vi "StageRotate.vi"(0 "Axis":T1={"Serial port handle"="", "Axis"="", "Controller #"=0, "Min position"=0.0, "Max position"=0.0, "Min velocity"=0.0, "Max velocity"=0.0, "Firmware"="", "Device ID"=0, "Variable event"=refnum, "Variable ref"=refnum, "Resolution, usteps/step"=0, "Serial port semaphore"=refnum, "Joystick buttons"={"MinDir"=1, "MaxDir"=2, "MedSpeed"=5, "HighSpeed"=6}} {"Joystick buttons"."HighSpeed" min=1 max=25 step=1; "Joystick buttons"."MedSpeed" min=1 max=25 step=1; "Joystick buttons"."MaxDir" min=1 max=25 step=1; "Joystick buttons"."MinDir" min=1 max=25 step=1}, 2 "Joystick event":T4, 3 "Stop event":refnum<user-event>, 5 "error in":errorcluster={"status"=FALSE, "code"=1073676294, "source"="VISA Read in Zaber TLCM.lvclass:Command.vi:1820008->Zaber TLCM.lvclass:Get home position.vi->Zaber TLCM.lvclass:Get limits.vi->Zaber TLCM.lvclass:Join.vi->Swan probe.vi"}) -> (14 "Axis out":T1={"Serial port handle"="", "Axis"="", "Controller #"=0, "Min position"=0.0, "Max position"=0.0, "Min velocity"=0.0, "Max velocity"=0.0, "Firmware"="", "Device ID"=0, "Variable event"=refnum, "Variable ref"=refnum, "Resolution, usteps/step"=0, "Serial port semaphore"=refnum, "Joystick buttons"={"MinDir"=1, "MaxDir"=2, "MedSpeed"=5, "HighSpeed"=6}} {"Joystick buttons"."HighSpeed" min=1 max=25 step=1; "Joystick buttons"."MedSpeed" min=1 max=25 step=1; "Joystick buttons"."MaxDir" min=1 max=25 step=1; "Joystick buttons"."MinDir" min=1 max=25 step=1}, 19 "error out":errorcluster)   [LabVIEW 2017]
uses:
  Joystick events/Joystick event.ctl
  GenericDataEvent/GenericEvent.ctl
  Zaber.ctl
  ZaberVariables.ctl
panel:
  out "JoystickValue":i16
  in  "Readback loop":bool
  in  "JoyHighVelocity":i32=6 caption="Max direction" min=1 max=25 step=1
  in  "JoyMediumVelocity":i32=5 caption="Max direction" min=1 max=25 step=1
  in  "JoyMaxDirection":i32=2 caption="Max direction" min=1 max=25 step=1
  in  "JoyMinDirection":i32=1 caption="Min direction" min=1 max=25 step=1
  in  "JoyHighVel":dbl=3.0 caption="High velocity, deg/s" min=1e-07 max=25.0 step=0.01 format="%#.4f"
  in  "JoyMediumVel":dbl=1.0 caption="Medium velocity, deg/s" min=1e-07 max=25.0 step=0.01 format="%#.4f"
  in  "JoyLowVel":dbl=0.02 caption="Low velocity, deg/s" min=1e-07 max=25.0 step=0.01 format="%#.4f"
  out "Name":string
  in  "VelocitySp":dbl=0.19998779296875002 caption="Velocity, deg/s" min=0.0 max=25.40003175 format="%#.6f"
  out "VelocityRb":dbl=0.19998779296875002 caption="X position" min=0.0 max=25.0 format="%#.6f"
  in  "PositionSp":dbl caption="Position, deg" min=0.0 max=25.40003175 format="%#.6f"
  in  "MaxSoftPosition":dbl=101.60003175000001 caption="Max soft position, deg" min=0.0 max=25.40003175 format="%#.4f"
  in  "MinSoftPosition":dbl caption="Min soft position, deg" min=0.0 max=25.40003175 format="%#.4f"
  out "PositionRb":dbl=0.8111490000000001 caption="X position" min=0.0 max=25.0 format="%#.6f"
  out "MaxVelocity":dbl=26.0 caption="Max velocity, deg/s" format="%#.4f"
  out "MaxPositionRb":dbl=101.60003175000001 caption="Max position, deg" format="%#.4f"
  out "MinPositionRb":dbl caption="Min position, deg" format="%#.4f"
  # "Joystick"
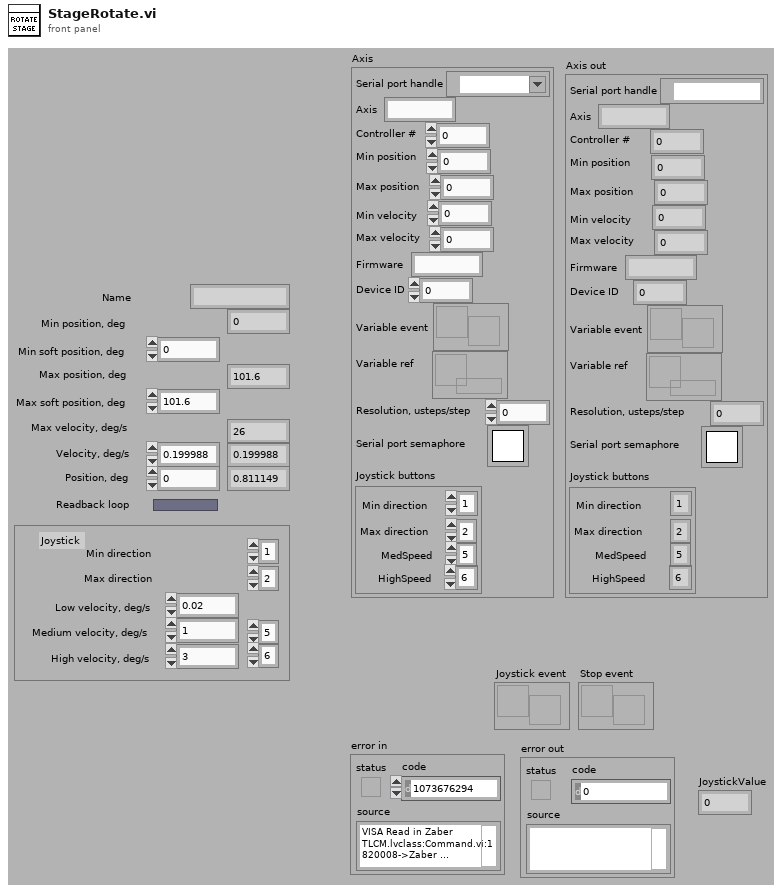
[diagram p1: front panel]
types:
  T1 = typedef "Zaber.ctl" = cluster{"Serial port handle":refnum<visa-resource-name>, "Axis":string, "Controller #":u8, "Min position":dbl, "Max position":dbl, "Min velocity":dbl, "Max velocity":dbl, "Firmware":string, "Device ID":i32, "Variable event":T2, "Variable ref":refnum<data-value>, "Resolution, usteps/step":i32, "Serial port semaphore":T3, "Joystick buttons":cluster{"MinDir":i32, "MaxDir":i32, "MedSpeed":i32, "HighSpeed":i32}}
  T2 = typedef "GenericEvent.ctl" = refnum<user-event>
  T3 = typedef "Semaphore RefNum" = refnum<k1>
  T4 = typedef "Joystick event.ctl" = refnum<user-event>
  T5 = cluster{"MinDir":i32, "MaxDir":i32, "MedSpeed":i32, "HighSpeed":i32}
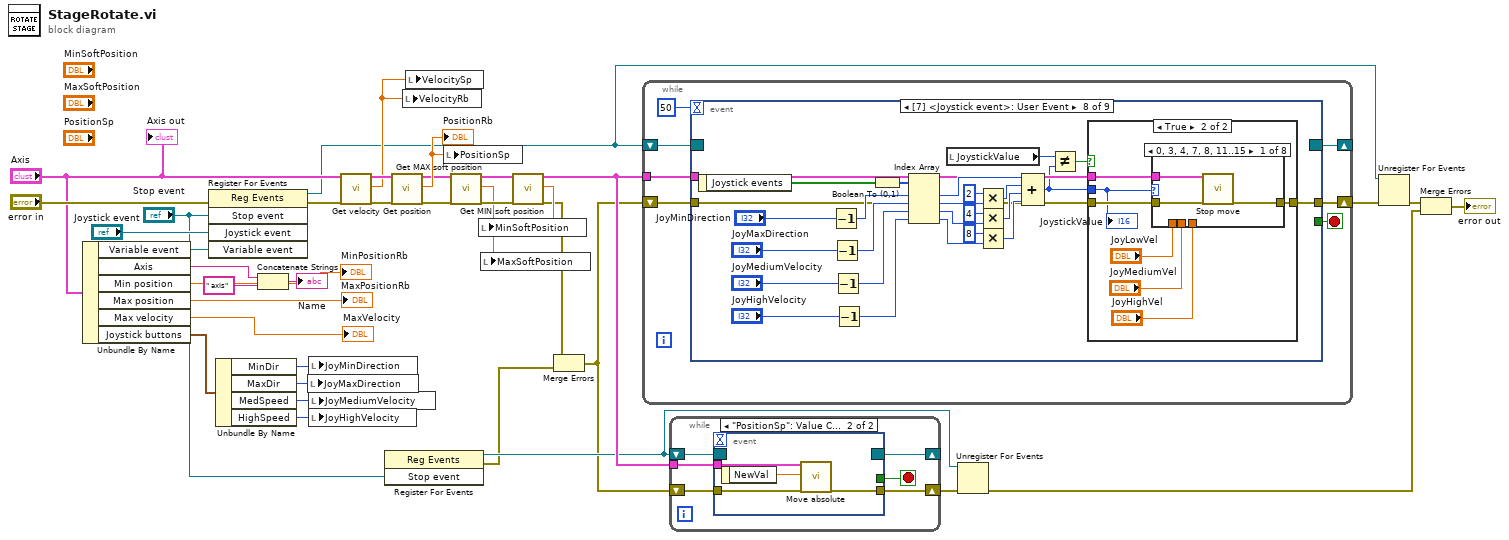
[diagram p0: block diagram]
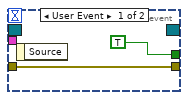
[diagram p2: hidden frame]
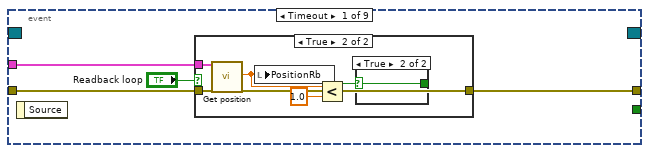
[diagram p3: hidden frame]
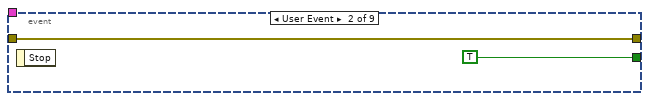
[diagram p6: hidden frame]
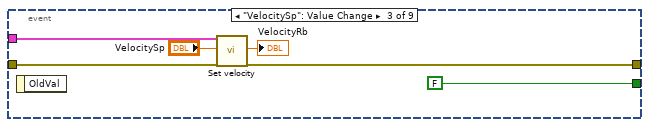
[diagram p7: hidden frame]
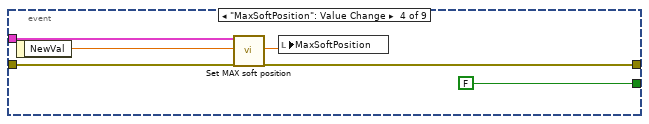
[diagram p8: hidden frame]
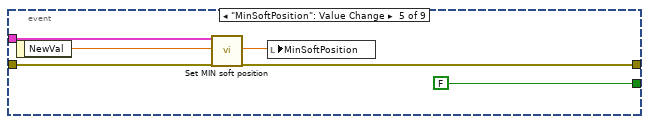
[diagram p9: hidden frame]
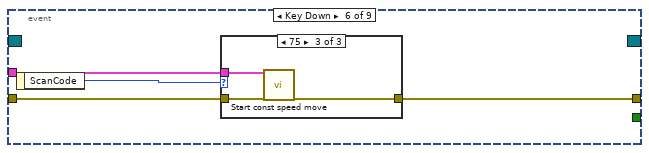
[diagram p10: hidden frame]
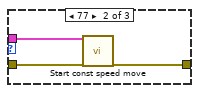
[diagram p12: hidden frame]
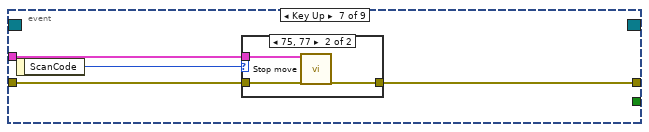
[diagram p13: hidden frame]
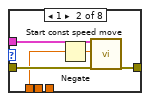
[diagram p16: hidden frame]
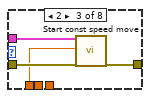
[diagram p17: hidden frame]
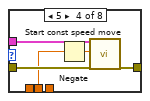
[diagram p18: hidden frame]
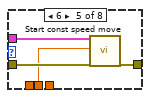
[diagram p19: hidden frame]
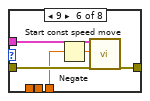
[diagram p20: hidden frame]
diagram:
  n1 = Unbundle By Name("Axis") -> ("Variable event"=w35:T2, "Axis"=w33:string, "Min position"=→"MinPositionRb":dbl, "Max position"=→"MaxPositionRb":dbl, "Max velocity"=→"MaxVelocity":dbl, "Joystick buttons"=w1:T5)
  n2 = register-events(error in="error in", "Stop event", "Joystick event", w35) -> (reference out=w11:refnum<event-registration>, error out=w27:errorcluster)  [unwired: 1 in]
  n3 = Unbundle By Name(w1) -> ("MinDir"=w16:i32, "MaxDir"=w15:i32, "MedSpeed"=w14:i32, "HighSpeed"=w13:i32)
  n4 = Concatenate Strings(w33, " axis" ("string")) -> (→"Name":string)
  n5 = local write "JoyMaxDirection"(w15) -> ()
  n6 = local write "JoyMinDirection"(w16) -> ()
  n7 = local write "JoyMediumVelocity"(w14) -> ()
  n8 = local write "JoyHighVelocity"(w13) -> ()
  n9 = call "Get velocity.vi"("Zaber"="Axis", "error in"=w27) -> ("Zaber out"=w31:T1, "Velocity, mm/s"=w30:dbl, "error out"=w38:errorcluster)  [unwired: 14 in, 1 out]
  n10 = register-events("Stop event") -> (reference out=w9:refnum<event-registration>, error out=w4:errorcluster)  [unwired: 2 in]
  n11 = call "Get position.vi"("Zaber"=w31, "error in"=w38) -> ("Zaber out"=w20:T1, "PositionRb"=w29:dbl, "error out"=w21:errorcluster)  [unwired: 13 in, 2 out]
  "PositionRb" <- w29
  n12 = local write "VelocityRb"(w30) -> ()
  n13 = local write "VelocitySp"(w30) -> ()
  n14 = local write "PositionSp"(w29) -> ()
  n15 = call "Get MAX soft position.vi"("Zaber"=w20, "error in"=w21) -> ("Zaber out"=w22:T1, "Max soft position"=w18:dbl, "error out"=w23:errorcluster)  [unwired: 15 in]
  n16 = local write "MaxSoftPosition"(w18) -> ()
  n17 = call "Get MIN soft position.vi"("Zaber"=w22, "error in"=w23) -> ("Zaber out"=w19:T1, "Min soft position"=w17:dbl, "error out"=w2:errorcluster)  [unwired: 15 in]
  n18 = local write "MinSoftPosition"(w17) -> ()
  n19 = Merge Errors(w2, w4) -> (w3:errorcluster)
  n20 = while {
    shift-right: [w42] -> w8
    shift-left: w3 -> [w43]
    tunnel: w19 -> [w44]
    shift-right: [w39] -> _
    shift-left: w11 -> [w41]
    stop <- w45 stop-if-true
    n21 = event shown="[7] <Joystick event>: User Event" {
      selector: w41 -> [_ _ _ _ _ _ _ _ _]
      dyn-events: [_ _ _ _ _ _ _ _ _] -> w39
      timeout: 50 -> [_ _ _ _ _ _ _ _ _]
      tunnel: [_ TRUE ("Stop") FALSE ("Stop") FALSE FALSE _ _ _ _] -> w45
      tunnel: w43 -> [w48 w59 w65 w70 w76 w80 w90 w103 w165]
      tunnel: w44 -> [w46 _ w60 w66 w72 w81 w91 w102 _]
      tunnel: [w47 w59 w62 w67 w74 w79 w89 w104 w162] -> w42
      event Timeout {
        n22 = event-data() -> ()  [unwired: 2 out]
        n23 = case shown="True" "Readback loop" {
          tunnel: w48 -> [w50 w56]
          tunnel: w46 -> [_ w54]
          tunnel: [w50 w55] -> w47
          frame False {
          }
          frame True {
            n24 = call "Get position.vi"("Zaber"=w54, "error in"=w56) -> ("PositionRb"=w53:dbl, "error out"=w55:errorcluster)  [unwired: 13 in, 3 out]
            n25 = local write "PositionRb"(w53) -> ()
            n26 = Less?(x=w53, y=1.0) -> (x < y?=w51:bool)
            n27 = case shown="True" w51 {
              selector: w51 -> [_ w57]
              tunnel: [_ w57] -> _
              frame False {
              }
              frame True {
              }
            }
          }
        }
      }
      event User Event {
        n28 = event-data() -> ()  [unwired: 2 out]
      }
      event "VelocitySp": Value Change {
        n29 = event-data() -> ()  [unwired: 2 out]
        n30 = call "Set velocity.vi"("Zaber in"=w60, "Velocity, mm/s"="VelocitySp", "error in"=w65) -> ("Velocity, mm/s"=→"VelocityRb":dbl, "error out"=w62:errorcluster)  [unwired: 14 in, 1 out]
      }
      event "MaxSoftPosition": Value Change {
        n31 = event-data() -> ("NewVal"=w69:dbl)  [unwired: 1 out]
        n32 = call "Set MAX soft position.vi"("Zaber"=w66, "Max soft position"=w69, "error in"=w70) -> ("Max soft position"=w68:dbl, "error out"=w67:errorcluster)  [unwired: 14 in, 1 out]
        n33 = local write "MaxSoftPosition"(w68) -> ()
      }
      event "MinSoftPosition": Value Change {
        n34 = event-data() -> ("NewVal"=w77:dbl)  [unwired: 1 out]
        n35 = call "Set MIN soft position.vi"("Zaber"=w72, "Min soft position"=w77, "error in"=w76) -> ("Min soft position"=w73:dbl, "error out"=w74:errorcluster)  [unwired: 14 in, 1 out]
        n36 = local write "MinSoftPosition"(w73) -> ()
      }
      event Key Down {
        n37 = event-data() -> ("ScanCode"=w78:i16)  [unwired: 1 out]
        n38 = case shown="75" w78 {
          tunnel: w81 -> [_ w85 w88]
          tunnel: w80 -> [w82 w84 w87]
          tunnel: [w82 w83 w86] -> w79
          frame 0, Default {
          }
          frame 77 {
            n39 = call "Start const speed move.vi"("Zaber"=w85, "error in"=w84) -> ("error out"=w83:errorcluster)  [unwired: 15 in, 2 out]
          }
          frame 75 {
            n40 = call "Start const speed move.vi"("Zaber"=w88, "error in"=w87) -> ("error out"=w86:errorcluster)  [unwired: 15 in, 2 out]
          }
        }
      }
      event Key Up {
        n41 = event-data() -> ("ScanCode"=w92:i16)  [unwired: 1 out]
        n42 = case shown="75, 77" w92 {
          tunnel: w91 -> [_ w96]
          tunnel: w90 -> [w93 w95]
          tunnel: [w93 w94] -> w89
          frame 0, Default {
          }
          frame 75, 77 {
            n43 = call "Stop move.vi"("Zaber"=w96, "error in"=w95) -> ("error out"=w94:errorcluster)  [unwired: 16 in, 1 out]
          }
        }
      }
      event User Event {
        n44 = event-data() -> ("Joystick events"=w122:bool[])  [unwired: 1 out]
        n45 = Decrement(x="JoyMinDirection") -> (x-1=w120:i32)
        n46 = Decrement(x="JoyMaxDirection") -> (x-1=w119:i32)
        n47 = Decrement(x="JoyMediumVelocity") -> (x-1=w118:i32)
        n48 = Decrement(x="JoyHighVelocity") -> (x-1=w117:i32)
        n49 = Boolean To (0,1)(Boolean=w122) -> (0, 1=w121:i16[])
        n50 = Index Array(array=w121, index #1=w120, index #2=w119, index #3=w118, index #4=w117) -> (element #1=w110:i16, element #2=w109:i16, element #3=w108:i16, element #4=w107:i16)
        n51 = local read "JoystickValue"() -> (w106:i16)
        n52 = Multiply(x=i16 2 ("y"), y=w109) -> (x*y=w113:i16)
        n53 = Multiply(x=i16 4 ("y"), y=w108) -> (x*y=w112:i16)
        n54 = Multiply(x=i16 8 ("y"), y=w107) -> (x*y=w111:i16)
        n55 = Compound Arithmetic op=ADD(w110, w113, w112, w111) -> (w101:i16)
        n56 = Not Equal?(x=w106, y=w101) -> (x != y?=w105:bool)
        n57 = case shown="True" w105 {
          tunnel: [w123 w130] -> w104
          tunnel: w103 -> [w123 w129]
          tunnel: w102 -> [_ w128]
          tunnel: w101 -> [_ w124]
          frame False {
          }
          frame True {
            n58 = case shown="0, 3, 4, 7, 8, 11..15" w124 {
              tunnel: w129 -> [w133 w136 w140 w145 w149 w154 w158 w161]
              tunnel: w128 -> [w132 w137 w141 w146 w150 w155 w159 _]
              tunnel: [w131 w138 w142 w147 w151 w156 w160 w161] -> w130
              tunnel: "JoyLowVel" -> [_ w134 w139 _ _ _ _ _]
              tunnel: "JoyMediumVel" -> [_ _ _ w143 w148 _ _ _]
              tunnel: "JoyHighVel" -> [_ _ _ _ _ w152 w157 _]
              frame 0, 3, 4, 7, 8, 11..15 {
                n59 = call "Stop move.vi"("Zaber"=w132, "error in"=w133) -> ("error out"=w131:errorcluster)  [unwired: 16 in, 1 out]
              }
              frame 1 {
                n60 = Negate(x=w134) -> (-x=w135:dbl)
                n61 = call "Start const speed move.vi"("Zaber"=w137, "Velocity, mm/s"=w135, "error in"=w136) -> ("error out"=w138:errorcluster)  [unwired: 14 in, 2 out]
              }
              frame 2 {
                n62 = call "Start const speed move.vi"("Zaber"=w141, "Velocity, mm/s"=w139, "error in"=w140) -> ("error out"=w142:errorcluster)  [unwired: 14 in, 2 out]
              }
              frame 5 {
                n63 = Negate(x=w143) -> (-x=w144:dbl)
                n64 = call "Start const speed move.vi"("Zaber"=w146, "Velocity, mm/s"=w144, "error in"=w145) -> ("error out"=w147:errorcluster)  [unwired: 14 in, 2 out]
              }
              frame 6 {
                n65 = call "Start const speed move.vi"("Zaber"=w150, "Velocity, mm/s"=w148, "error in"=w149) -> ("error out"=w151:errorcluster)  [unwired: 14 in, 2 out]
              }
              frame 9 {
                n66 = Negate(x=w152) -> (-x=w153:dbl)
                n67 = call "Start const speed move.vi"("Zaber"=w155, "Velocity, mm/s"=w153, "error in"=w154) -> ("error out"=w156:errorcluster)  [unwired: 14 in, 2 out]
              }
              frame 10 {
                n68 = call "Start const speed move.vi"("Zaber"=w159, "Velocity, mm/s"=w157, "error in"=w158) -> ("error out"=w160:errorcluster)  [unwired: 14 in, 2 out]
              }
              frame Default {
              }
            }
            "JoystickValue" <- w124
          }
        }
      }
      event User Event {
        n69 = event-data() -> ("Name"=w164:string, "Variant"=w163:variant)  [unwired: 1 out]
        n70 = case shown="\"Speed\"" w164 {
          tunnel: w163 -> [_ w170 w173]
          tunnel: w165 -> [w166 w169 w174]
          tunnel: [w166 w168 w172] -> w162
          frame Default {
          }
          frame "Position" {
            n71 = Variant To Data(error in=w169, Variant=w170) -> (data=w167:dbl, error out=w168:errorcluster)  [unwired: 1 in]
            n72 = local write "PositionRb"(w167) -> ()
          }
          frame "Speed" {
            n73 = Variant To Data(error in=w174, Variant=w173) -> (data=w171:dbl, error out=w172:errorcluster)  [unwired: 1 in]
            n74 = local write "VelocityRb"(w171) -> ()
          }
        }
      }
    }
  }
  n75 = while {
    shift-right: [w179] -> w10
    shift-left: w3 -> [w180]
    tunnel: w19 -> [w178]
    shift-right: [w175] -> _
    shift-left: w9 -> [w177]
    stop <- w176 stop-if-true
    n76 = event shown="[1] \"PositionSp\": Value Change" {
      selector: w177 -> [_ _]
      dyn-events: [_ _] -> w175
      timeout: _ -> [_ _]
      tunnel: w180 -> [w181 w186]
      tunnel: [w181 w183] -> w179
      tunnel: w178 -> [_ w185]
      tunnel: [TRUE ("Stop") _] -> w176
      event User Event {
        n77 = event-data() -> ()  [unwired: 1 in, 1 out]
      }
      event "PositionSp": Value Change {
        n78 = event-data() -> ("NewVal"=w184:dbl)  [unwired: 1 in]
        n79 = call "Move absolute.vi"("Zaber"=w185, "Position, mm"=w184, "error in"=w186) -> ("error out"=w183:errorcluster)  [unwired: 13 in, 3 out]
      }
    }
  }
  n80 = Unregister For Events(event registration refnum=w9, error in=w10) -> (error out=w7:errorcluster)
  n81 = Unregister For Events(event registration refnum=w11, error in=w8) -> (error out=w6:errorcluster)
  n82 = Merge Errors(w6, w7) -> (→"error out":errorcluster)
  "Axis out" <- "Axis"
